vi "Stop Core.vi"(10 "final error code":i32, 11 "DAQ Device in":refnum<class "DAQ Device.lvclass">) -> (3 "DAQ Device out":refnum<class "DAQ Device.lvclass">)   [LabVIEW 2014, in "DAQ Device.lvclass"]
doc: "(<B>Filename</B>: Actor Framework.lvlib:Actor.lvclass:Stop Core.vi)\n\nDefines what the actor does before it stops. Use the <B>final error code</B> input to determine whether the actor shut down in response to an error.\n\nBy default, this method does nothing. A descendant class may override it to define behavior, such as shutting down any processes the actor initiated in its override of the Actor Core method."
uses:
  DAQ Device.lvclass
  DAQ Device.lvclass/DAQ Device.ctl
  Session APIs/Session Log/System Log.lvclass
  <vilib>/ActorFramework/Actor/Actor.lvclass
  <userlib>/_Session Fwk/Session - Root.lvclass
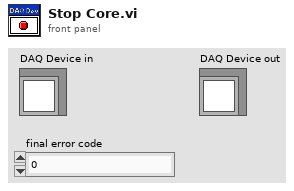
[diagram p1: front panel]
types:
  T1 = typedef "Session - Root.lvclass/Session Handle.ctl" = refnum<data-value>
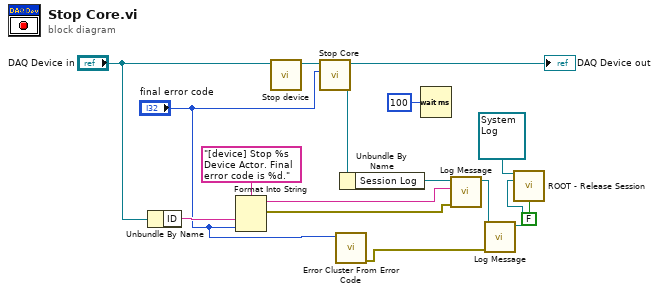
[diagram p0: block diagram]
diagram:
  n1 = Unbundle By Name("DAQ Device in") -> ("ID"=w9:string)
  n2 = Format Into String(format string="[device] Stop %s Device Actor. Final error code is %d.", w9, "final error code") -> (resulting string=w7:string, error out=w6:errorcluster)  [unwired: 2 in]
  n3 = call-dynamic "Stop device.vi"("DAQ Device in"="DAQ Device in") -> ("DAQ Device out"=w15:refnum<class "DAQ Device.lvclass">)  [unwired: 9 in, 1 out]
  n4 = call-parent "Stop Core.vi"("final error code"="final error code", "Actor in"=w15) -> ("Actor out"=w14:refnum<class "DAQ Device.lvclass">)  [unwired: 9 in]
  "DAQ Device out" <- w14
  n5 = call <vilib>:"Error Cluster From Error Code.vi"("error code (0)"="final error code") -> ("error out"=w3:errorcluster)  [unwired: 8 in]
  n6 = Unbundle By Name(w14) -> ("Session Log"=w11:T1)
  n7 = Wait (ms)(milliseconds to wait=u32 100) -> ()  [unwired: 1 out]
  n8 = call "Log Message.vi"("error in"=w6, "MSG In"=w7, "session in"=w11) -> ("session out"=w5:T1)  [unwired: 7 in, 1 out]
  n9 = call "Log Message.vi"("error in"=w3, "session in"=w5) -> ("session out"=w2:T1)  [unwired: 8 in, 1 out]
  n10 = call <userlib>:"ROOT - Release Session.vi"("OBJ - Session in"=refnum<class "System Log.lvclass"> refnum ("Sys Log"), "Session Handle in"=w2, "force destroy? (F)"=FALSE) -> ()  [unwired: 11 in, 2 out]
